vi "getPortIP.vi"(3 "error in (no error)":errorcluster, 5 "VISA resource name":refnum<visa-resource-name>="COM1" caption="PortIn") -> (0 "error out":errorcluster, 1 "portIP":string, 2 "VISA resource name 2":refnum<visa-resource-name>="COM1" caption="PortOut")   [LabVIEW 2010]
uses:
  GlobalCostants.vi
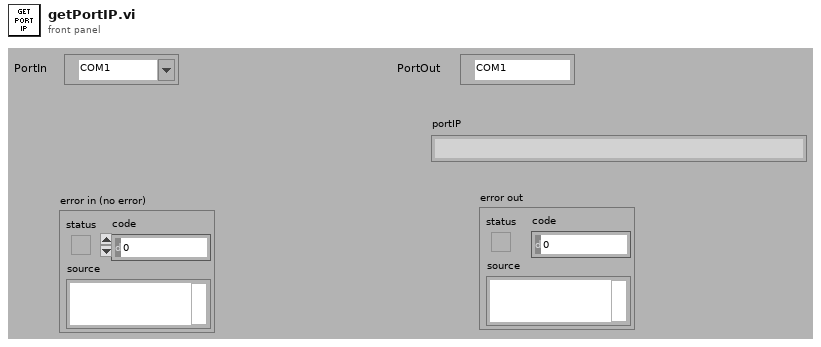
[diagram p1: front panel]
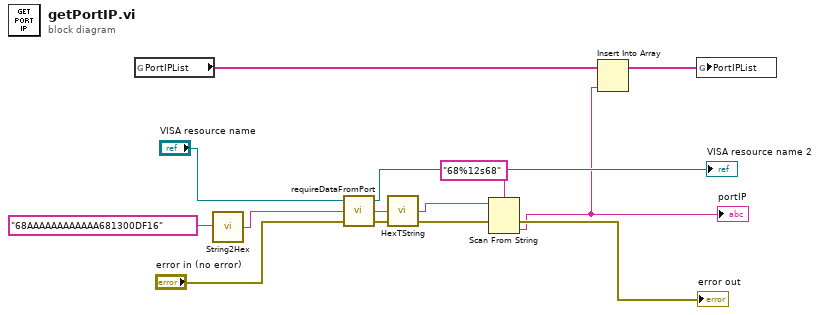
[diagram p0: block diagram]
diagram:
  n1 = global read "GlobalCostants.vi" "PortIPList"() -> (w6:string[])
  n2 = call "String2Hex.vi"("value"="68AAAAAAAAAAAA681300DF16") -> ("String"=w7:string)
  n3 = call "requireDataFromPort.vi"("error in (no error)"="error in (no error)", "Command"=w7, "VISA resource name"="VISA resource name") -> ("error out"=→"error out":errorcluster, "Data"=w4:string, "VISA resource name 2"=→"VISA resource name 2":refnum<visa-resource-name>)
  n4 = call "HexTString.vi"("input Hex"=w4) -> ("output string"=w3:string)
  n5 = Scan From String(format string="68%12s68" ("格式字符串"), input string=w3) -> (output 1=w1:string)  [unwired: 3 in, 3 out]
  "portIP" <- w1
  n6 = Insert Into Array(array=w6, new element=w1) -> (w5:string[])  [unwired: 1 in]
  n7 = global write "GlobalCostants.vi" "PortIPList"(w5) -> ()
